vi "Decompose Array.vi"(8 "error in (no error)":errorcluster, 11 "Variant Array":variant) -> (0 "error out":errorcluster, 1 "Dimension Sizes":i32[](array[numeric]), 2 "Elements":variant[](array[variant]), 3 "Size":i32)   [LabVIEW 2017, in "Composition.lvlib"]
doc: "Decomposes a Variant Array of any number of dimensions into its elements."
uses:
  Composition.lvlib
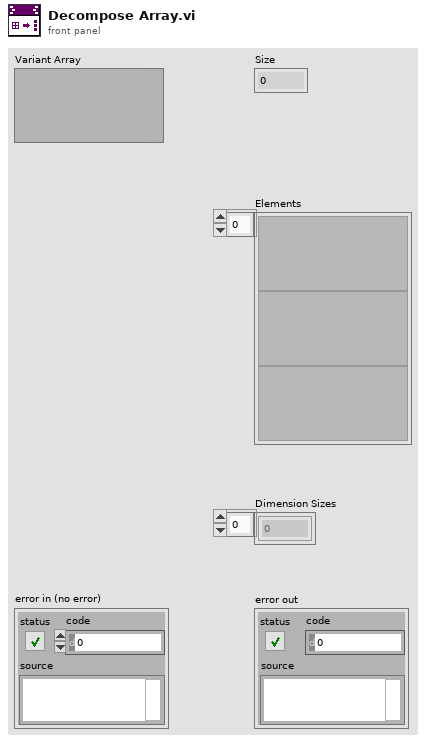
[diagram p1: front panel]
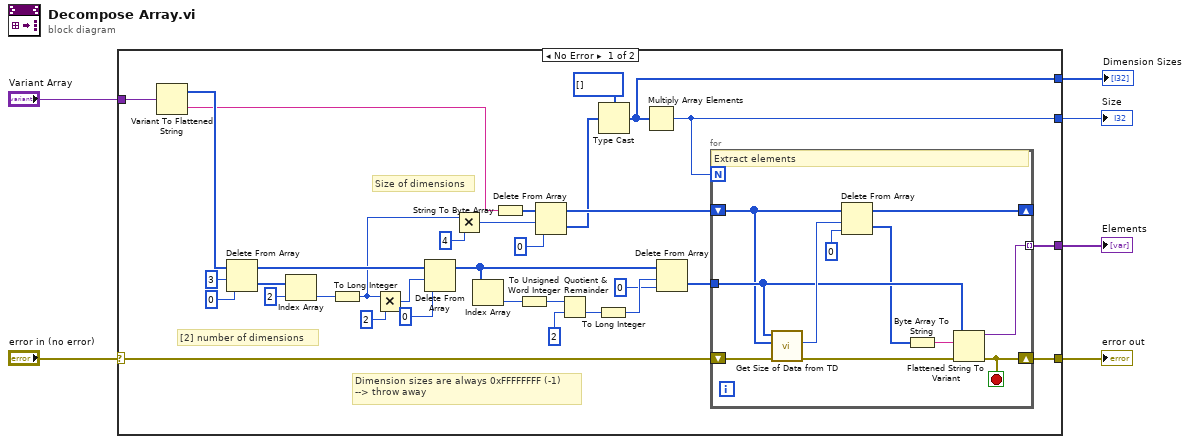
[diagram p0: block diagram]
diagram:
  n1 = case shown="No Error" "error in (no error)" {
    selector: "error in (no error)" -> [w35 w51]
    tunnel: [w38 _] -> w6
    tunnel: "Variant Array" -> [w37 _]
    tunnel: [w36 w51] -> w4
    tunnel: [w8 _] -> w3
    tunnel: [w7 _] -> w1
    frame No Error {
      # "Size of dimensions"
      # "Dimension sizes are always 0xFFFFFFFF (-1)\n--> throw away"
      # "[2] number of dimensions"
      n2 = Variant To Flattened String(Variant=w37) -> (data string=w16:string, 1:w34:i16[])
      n3 = Delete From Array(array=w34, length=3, index=0) -> (deleted portion=w24:i16[], array with subset deleted=w20:i16[])
      n4 = Index Array(array=w24, index=2) -> (element=w22:i16)
      n5 = To Long Integer(number=w22) -> (32bit integer=w11:i32)
      n6 = Multiply(x=w11, y=2) -> (x*y=w18:i32)
      n7 = Delete From Array(array=w20, length=w18, index=0) -> (array with subset deleted=w19:i16[])  [unwired: 1 out]
      n8 = Multiply(x=w11, y=4) -> (x*y=w12:i32)
      n9 = Index Array(array=w19) -> (element=w31:i16)  [unwired: 1 in]
      n10 = String To Byte Array(string=w16) -> (unsigned byte array=w15:u8[])
      n11 = To Unsigned Word Integer(number=w31) -> (unsigned 16bit integer=w29:u16)
      n12 = Delete From Array(array=w15, length=w12, index=0) -> (deleted portion=w9:u8[], array with subset deleted=w10:u8[])
      n13 = Quotient & Remainder(x=w29, y=u16 2) -> (floor(x/y)=w28:u16)  [unwired: 1 out]
      n14 = To Long Integer(number=w28) -> (32bit integer=w27:i32)
      n15 = Type Cast(type=i32[] [], x=w9) -> (*(type *) &x=w7:i32[])
      n16 = Multiply Array Elements(1:w7) -> (0:w8:i32)
      n17 = Delete From Array(array=w19, length=w27, index=0) -> (deleted portion=w25:i16[])  [unwired: 1 out]
      n18 = for {
        N: w8 -> [_]
        shift-right: [w47] -> _
        shift-left: w10 -> [w41]
        tunnel: [w50] -> w38 mode=indexing
        shift-right: [w48] -> w36
        shift-left: w35 -> [w45]
        tunnel: w25 -> [w42]
        stop <- w48 stop-if-true
        # "Extract elements"
        n19 = call "Get Size of Data from TD.vi"("error in (no error)"=w45, "Data String"=w41, "Type Descriptor"=w42) -> ("error out"=w44:errorcluster, "Size of Data"=w43:i32)  [unwired: 7 in]
        n20 = Delete From Array(array=w41, length=w43, index=0) -> (deleted portion=w40:u8[], array with subset deleted=w47:u8[])
        n21 = Byte Array To String(unsigned byte array=w40) -> (string=w49:string)
        n22 = Flattened String To Variant(4:w44, 6:w49, 7:w42) -> (0:w48:errorcluster, 3:w50:variant)
      }
    }
    frame Error {
    }
  }
  "Size" <- w3
  "Elements" <- w6
  "error out" <- w4
  "Dimension Sizes" <- w1
